vi "Configure Voltage Parameters.vi"(0 "VISA resource name":refnum<visa-resource-name>, 1 "Measurement (1: Voltage Channel 1)":i32(ring)=1 items=["Voltage Channel 1"=1, "Voltage Channel 2"=2], 5 "Voltage Resolution (8)":i32=8, 7 "Range Value (12)":dbl=12.0, 9 "Autorange (T: Enable)":bool=TRUE, 11 "error in (no error)":errorcluster, 12 "Enable Ratio (F: Disable)":bool, 13 "Enable Delta (F: Disable)":bool) -> (4 "VISA resource name out":refnum<visa-resource-name>, 15 "error out":errorcluster)   [LabVIEW 2022 SP3, in "Keithley 2182.lvlib"]
doc: "Configures voltage measurements for the specified channel.\n\n<B>Note:</B>\nIn order to enable voltage measurements on a specific channel, use the <B>Configure Measurements</B> VI."
uses:
  <instrlib>/Keithley 2182/Keithley 2182.lvlib
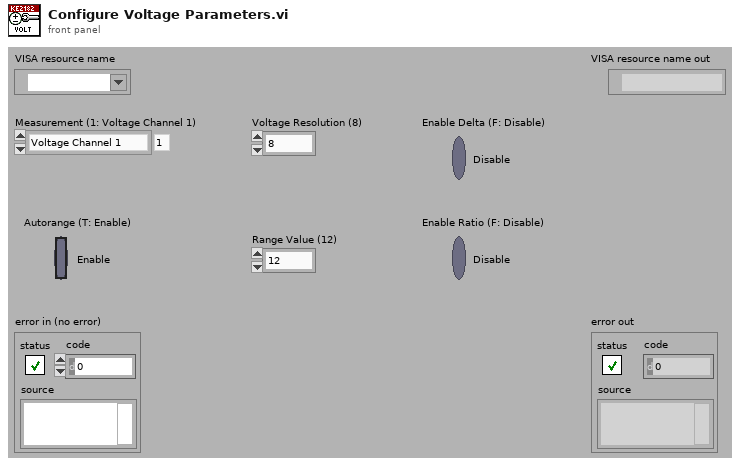
[diagram p1: front panel]
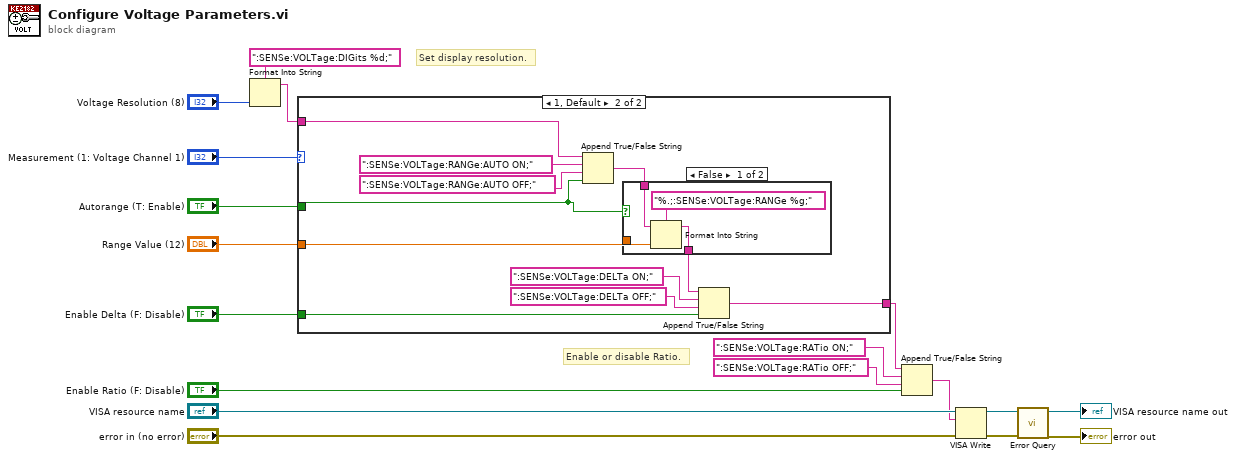
[diagram p0: block diagram]
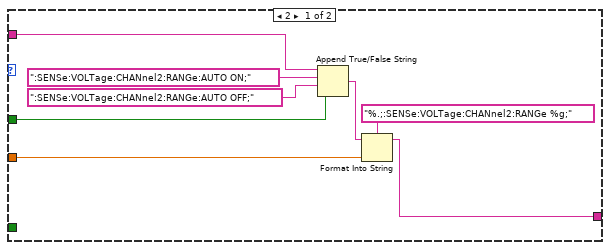
[diagram p2: hidden frame]
diagram:
  # "Enable or disable Ratio."
  # "Set display resolution."
  n1 = Format Into String "Format Into String"(format string=":SENSe:VOLTage:DIGits %d;", "Voltage Resolution (8)") -> (resulting string=w3:string)  [unwired: 2 in, 1 out]
  n2 = case shown="1, Default" "Measurement (1: Voltage Channel 1)" {
    tunnel: "Enable Delta (F: Disable)" -> [_ w30]
    tunnel: [w20 w35] -> w2
    tunnel: "Autorange (T: Enable)" -> [w23 w27]
    tunnel: "Range Value (12)" -> [w22 w32]
    tunnel: w3 -> [w19 w28]
    frame 2 {
      n3 = Append True/False String(1:w23, 2:":SENSe:VOLTage:CHANnel2:RANGe:AUTO OFF;", 3:":SENSe:VOLTage:CHANnel2:RANGe:AUTO ON;", 4:w19) -> (0:w21:string)
      n4 = Format Into String(format string="%.;:SENSe:VOLTage:CHANnel2:RANGe %g;", initial string=w21, w22) -> (resulting string=w20:string)  [unwired: 1 in, 1 out]
    }
    frame 1, Default {
      n5 = Append True/False String(1:w27, 2:":SENSe:VOLTage:RANGe:AUTO OFF;", 3:":SENSe:VOLTage:RANGe:AUTO ON;", 4:w28) -> (0:w31:string)
      n6 = case shown="False" w27 {
        tunnel: w32 -> [w40 _]
        tunnel: w31 -> [w39 w42]
        tunnel: [w38 w42] -> w29
        frame False {
          n7 = Format Into String "Format Into String"(format string="%.;:SENSe:VOLTage:RANGe %g;", initial string=w39, w40) -> (resulting string=w38:string)  [unwired: 1 in, 1 out]
        }
        frame True {
        }
      }
      n8 = Append True/False String(1:w30, 2:":SENSe:VOLTage:DELTa OFF;", 3:":SENSe:VOLTage:DELTa ON;", 4:w29) -> (0:w35:string)
    }
  }
  n9 = Append True/False String(1:"Enable Ratio (F: Disable)", 2:":SENSe:VOLTage:RATio OFF;", 3:":SENSe:VOLTage:RATio ON;", 4:w2) -> (0:w1:string)
  n10 = VISA Write(VISA resource name="VISA resource name", write buffer=w1, error in (no error)="error in (no error)") -> (VISA resource name out=w15:refnum<visa-resource-name>, error out=w14:errorcluster)  [unwired: 1 out]
  n11 = call <instrlib>:"Error Query.vi"("error in (no error)"=w14, "VISA resource name"=w15) -> ("error out"=→"error out":errorcluster, "VISA resource name out"=→"VISA resource name out":refnum<visa-resource-name>)  [unwired: 6 in, 2 out]
